vi "Target Init Controller.vi"(8 "error in (no error)":errorcluster) -> (0 "error out":errorcluster)   [LabVIEW 2018]
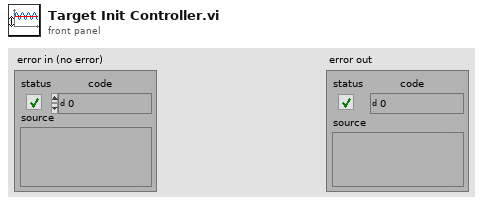
[diagram p1: front panel]
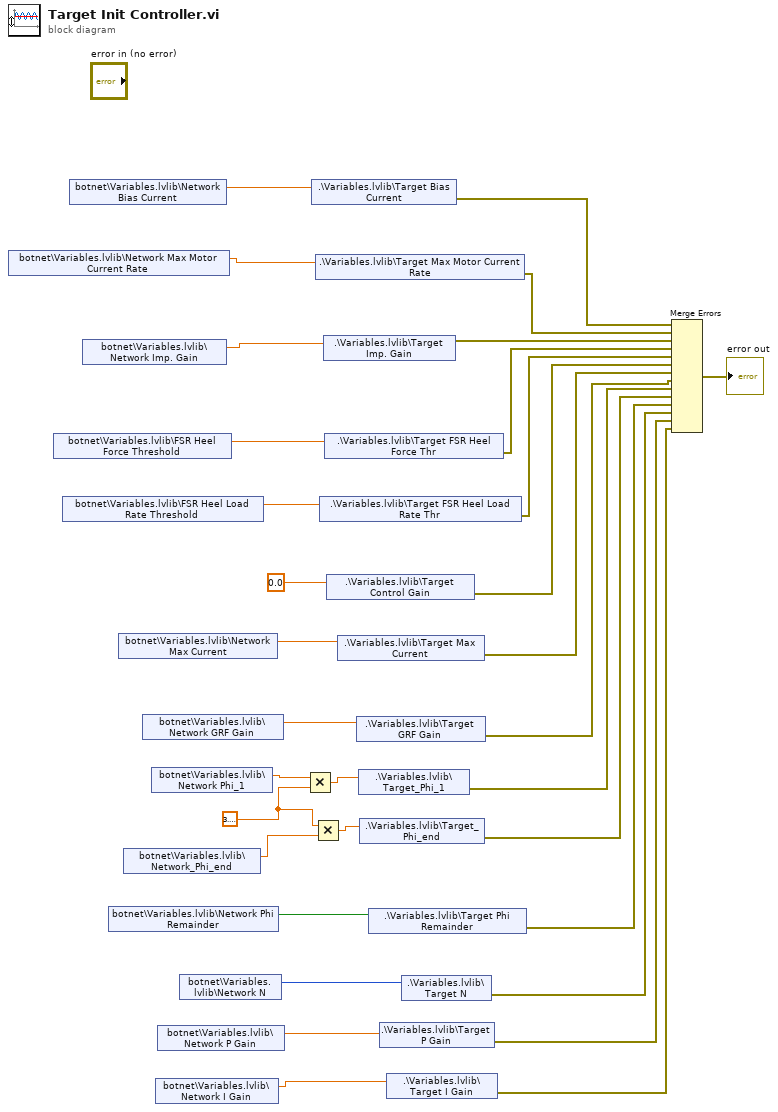
[diagram p0: block diagram]
diagram:
  w9 = 3.141592653589793
  n1 = shared-variable "botnet\\Variables.lvlib\\Network Max Motor Current Rate"() -> (w31:dbl)  [unwired: 1 in, 1 out]
  n2 = shared-variable "botnet\\Variables.lvlib\\FSR Heel Force Threshold"() -> (w29:dbl)  [unwired: 1 in, 1 out]
  n3 = shared-variable "botnet\\Variables.lvlib\\FSR Heel Load Rate Threshold"() -> (w28:dbl)  [unwired: 1 in, 1 out]
  n4 = shared-variable "botnet\\Variables.lvlib\\Network Bias Current"() -> (w32:dbl)  [unwired: 1 in, 1 out]
  n5 = shared-variable "botnet\\Variables.lvlib\\Network Imp. Gain"() -> (w30:dbl)  [unwired: 1 in, 1 out]
  n6 = shared-variable "botnet\\Variables.lvlib\\Network Phi Remainder"() -> (w7:bool)  [unwired: 1 in, 1 out]
  n7 = shared-variable "botnet\\Variables.lvlib\\Network Max Current"() -> (w26:dbl)  [unwired: 1 in, 1 out]
  n8 = shared-variable "botnet\\Variables.lvlib\\Network_Phi_end"() -> (w10:dbl)  [unwired: 1 in, 1 out]
  n9 = shared-variable "botnet\\Variables.lvlib\\Network GRF Gain"() -> (w17:dbl)  [unwired: 1 in, 1 out]
  n10 = shared-variable "botnet\\Variables.lvlib\\Network Phi_1"() -> (w13:dbl)  [unwired: 1 in, 1 out]
  n11 = shared-variable "botnet\\Variables.lvlib\\Network I Gain"() -> (w3:dbl)  [unwired: 1 in, 1 out]
  n12 = shared-variable "botnet\\Variables.lvlib\\Network P Gain"() -> (w4:dbl)  [unwired: 1 in, 1 out]
  n13 = shared-variable "botnet\\Variables.lvlib\\Network N"() -> (w6:u32)  [unwired: 1 in, 1 out]
  n14 = Multiply(x=w13, y=w9) -> (x*y=w12:dbl)
  n15 = shared-variable ".\\Variables.lvlib\\Target Bias Current"(w32) -> (error out=w25:errorcluster)  [unwired: 1 in]
  n16 = Multiply(x=w9, y=w10) -> (x*y=w11:dbl)
  n17 = shared-variable ".\\Variables.lvlib\\Target Max Motor Current Rate"(w31) -> (error out=w24:errorcluster)  [unwired: 1 in]
  n18 = shared-variable ".\\Variables.lvlib\\Target FSR Heel Load Rate Thr"(w28) -> (error out=w20:errorcluster)  [unwired: 1 in]
  n19 = shared-variable ".\\Variables.lvlib\\Target Imp. Gain"(w30) -> (error out=w22:errorcluster)  [unwired: 1 in]
  n20 = shared-variable ".\\Variables.lvlib\\Target FSR Heel Force Thr"(w29) -> (error out=w21:errorcluster)  [unwired: 1 in]
  n21 = shared-variable ".\\Variables.lvlib\\Target Control Gain"(0.0 ("Target Control Gain")) -> (error out=w19:errorcluster)  [unwired: 1 in]
  n22 = shared-variable ".\\Variables.lvlib\\Target Max Current"(w26) -> (error out=w18:errorcluster)  [unwired: 1 in]
  n23 = shared-variable ".\\Variables.lvlib\\Target GRF Gain"(w17) -> (error out=w16:errorcluster)  [unwired: 1 in]
  n24 = shared-variable ".\\Variables.lvlib\\Target_Phi_1"(w12) -> (error out=w15:errorcluster)  [unwired: 1 in]
  n25 = shared-variable ".\\Variables.lvlib\\Target_Phi_end"(w11) -> (error out=w14:errorcluster)  [unwired: 1 in]
  n26 = shared-variable ".\\Variables.lvlib\\Target Phi Remainder"(w7) -> (error out=w8:errorcluster)  [unwired: 1 in]
  n27 = shared-variable ".\\Variables.lvlib\\Target P Gain"(w4) -> (error out=w2:errorcluster)  [unwired: 1 in]
  n28 = shared-variable ".\\Variables.lvlib\\Target I Gain"(w3) -> (error out=w1:errorcluster)  [unwired: 1 in]
  n29 = shared-variable ".\\Variables.lvlib\\Target N"(w6) -> (error out=w5:errorcluster)  [unwired: 1 in]
  n30 = Merge Errors(w25, w24, w22, w21, w20, w19, w18, w16, w15, w14, w8, w5, w2, w1) -> (→"error out":errorcluster)
